vi "LTS60_TCP_init.vi"() -> (0 "error out":errorcluster, 2 "TCP Connected":bool, 3 "connection ID out":refnum<k5>)   [LabVIEW 2019]
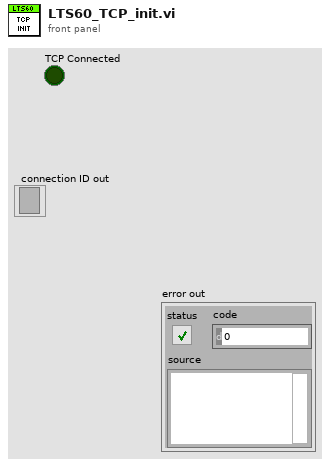
[diagram p1: front panel]
types:
  T1 = enum16{"Standard", "Buffered", "CRLF", "Immediate"}
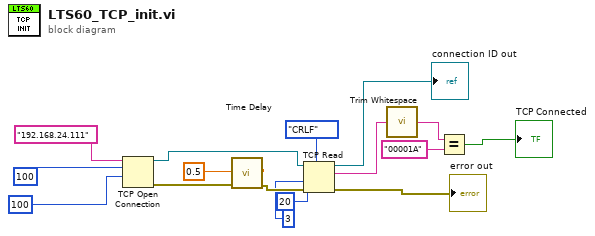
[diagram p0: block diagram]
diagram:
  n1 = TCP Open Connection(address="192.168.24.111", remote port or service name=u16 100, timeout ms (60000)=100) -> (connection ID=w11:refnum<k5>, error out=w16:errorcluster)  [unwired: 2 in]
  n2 = call "Time Delay"("error in (no error)"=w16, "Delay Time (s)"=0.5) -> ("error out"=w12:errorcluster)  [unwired: 9 in]
  n3 = TCP Read(connection ID=w11, bytes to read=20, error in (no error)=w12, 7:T1."CRLF" ("mode (standard)"), 9:3 ("timeout ms (25000)")) -> (connection ID out=→"connection ID out":refnum<k5>, data out=w4:string, error out=→"error out":errorcluster)
  n4 = call <vilib>:"Trim Whitespace.vi"("string"=w4) -> ("trimmed string"=w3:string)  [unwired: 1 in]
  n5 = Equal?(x=w3, y="00001A") -> (x = y?=→"TCP Connected":bool)
